vi "SPI IP.vi"() -> ()   [LabVIEW 2015]
uses:
  <userlib>/_NI SPI IP/FPGA/Controllers/Public/Transfer Settings.ctl
  <vilib>/Platform/TimedLoop/XDataNode/timing_clust.ctl
  <vilib>/Platform/TimedLoop/XDataNode/nitl_modes.ctl
  <vilib>/Platform/TimedLoop/XDataNode/wakeup.ctl
  <userlib>/_NI SPI IP/FPGA/Controllers/Public/Spi Master Inputs.ctl
  <vilib>/rvi/eio/common/nirviEmuTemplateMethod_errors.vi
  <vilib>/rvi/Emulation/niFpgaSctlEmulationGetInTimedLoop.vi
  <vilib>/rvi/Emulation/niFpgaEmulationReportErrorSimple.vi
  <vilib>/rvi/Emulation/niFpgaGetClockAttributes.vi
  <vilib>/rvi/Emulation/niFpgaCriticalErrorInLSC.vi
  SubVIs/Digital Logic/FPGA Simple PWM U32.vi
  <vilib>/eio/EIONode/EIONode.xnode
  <vilib>/Platform/TimedLoop/XDataNode/XDataNode.xnode
  <userlib>/_NI SPI IP/FPGA/Controllers/NI SPI IP FPGA.lvlib
  <vilib>/Platform/TimedLoop/XDataNode/XDNodeRunTimeDep.lvlib
panel:
  out "MOSI":bool
  out "Clock":bool
  out "Chip Select":bool
  in  "spi transfer settings":T1={"Divide Value"=20, "Transfer Length (bits)"=32, "CS Asserted Polarity"=FALSE, "Clock Polarity (CPOL)"=FALSE, "Clock Phase (CPHA)"=FALSE, "Lengthen MISO Setup"=FALSE, "Direction Change Bit"=0, "MOSI Starts as Output"=FALSE, "Tristatable MOSI"=FALSE} {"Direction Change Bit" max=64 step=1; "Transfer Length (bits)" min=1 max=64 step=1}
  in  "manual assert chip select":bool
  out "ready for input":bool
  out "read data":u64 format="%.0x"
  in  "data to write":u64 format="%.0x"
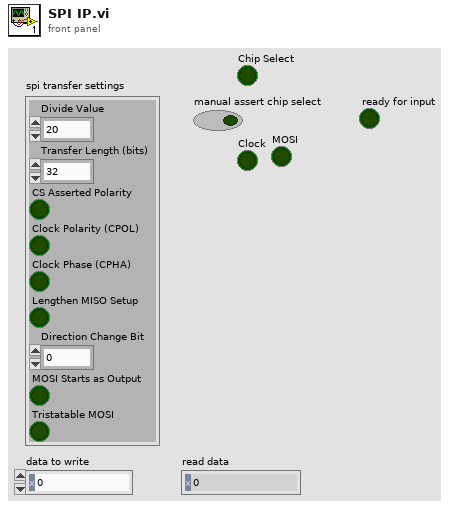
[diagram p1: front panel]
types:
  T1 = typedef "NI SPI IP FPGA.lvlib/Transfer Settings.ctl" = cluster{"Divide Value":u8, "Transfer Length (bits)":u8, "CS Asserted Polarity":bool, "Clock Polarity (CPOL)":bool, "Clock Phase (CPHA)":bool, "Lengthen MISO Setup":bool, "Direction Change Bit":u8, "MOSI Starts as Output":bool, "Tristatable MOSI":bool}
  T2 = typedef "NI SPI IP FPGA.lvlib/Spi Master Inputs.ctl" = cluster{"MISO":bool}
  T3 = typedef "XDNodeRunTimeDep.lvlib/timing_clust.ctl" = cluster{"Expected End [f-1]":u64, "Actual End [f-1]":u64, "Finished Late? [f-1]":bool, "Expected End [i-1]":u64, "Actual End [i-1]":u64, "Finished Late? [i-1]":bool, "Expected Start [i]":u64, "Actual Start [i]":u64, "Expected Start [f]":u64, "Actual Start [f]":u64, "Source Name":string, "Structure Name":string, "Period":i64, "Deadline":i64, "Offset":i64, "Start":i64, "Priority":i32, "Timeout":i32, "Mode":T4, "Wakeup Reason":T5, "Error":errorcluster, "Source Type":string, "Secondary Source Type":string, "Global End Time":u64, "Global Start Time":u64, "Frame Duration":u64, "Iteration Duration":u64, "Assigned CPU":i32, "I/O Scan Engine Mode":u32}
  T4 = typedef "XDNodeRunTimeDep.lvlib/nitl_modes.ctl" = enum32{"No Change", "Process missed periods, maintain original phase", "Discard missed periods, maintain original phase", "Process missed periods, ignore original phase", "Discard missed periods, ignore original phase"}
  T5 = typedef "XDNodeRunTimeDep.lvlib/wakeup.ctl" = enum32{"Normal", "Aborted", "Asynchronous wakeup", "Timing source error", "Timed loop error", "Timeout"}
  T6 = typedef "NI SPI IP FPGA.lvlib/Spi Master Outputs.ctl" = cluster{"Chip Select":bool, "Clock":bool, "MOSI":bool, "MOSI OE":bool}
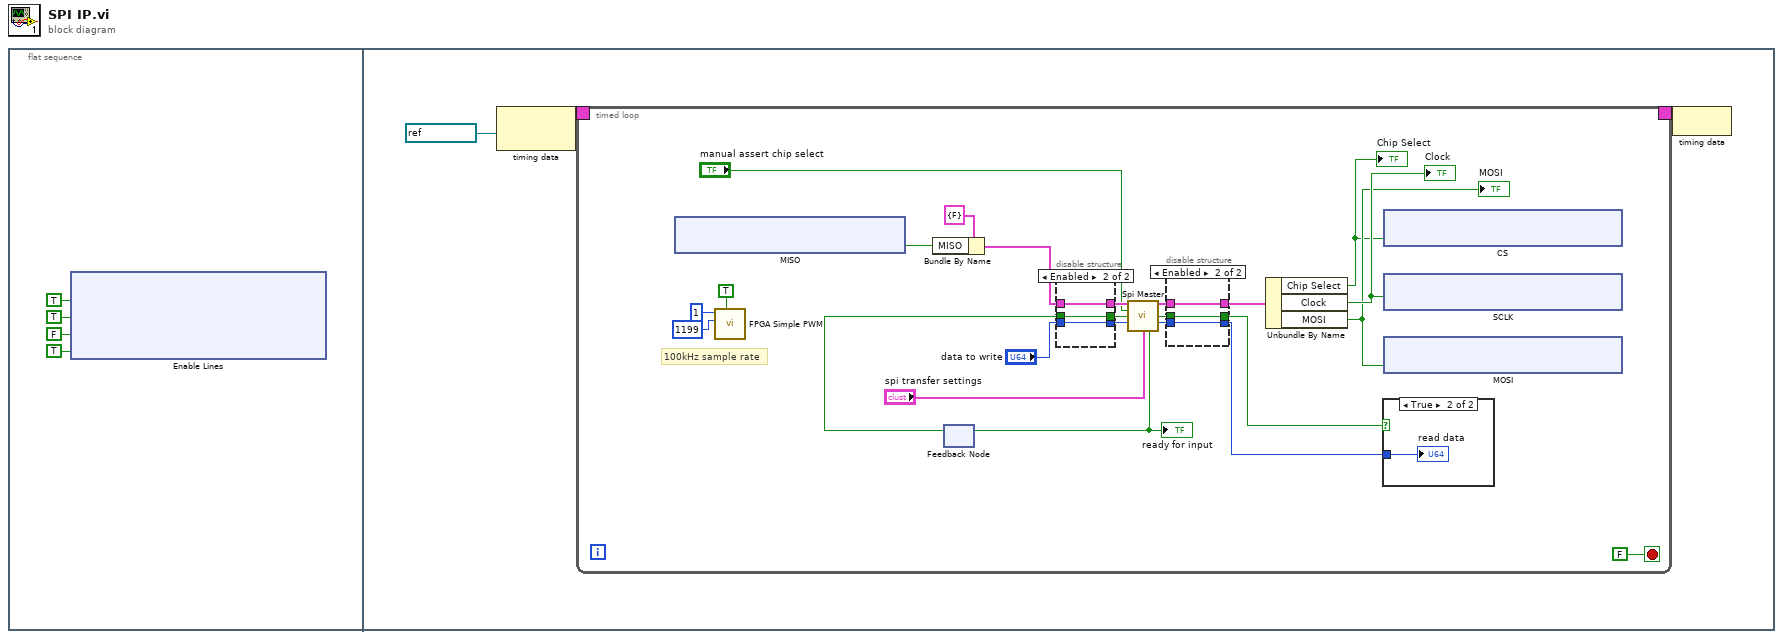
[diagram p0: block diagram]
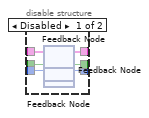
[diagram p2: hidden frame]
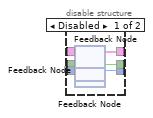
[diagram p3: hidden frame]
diagram:
  n1 = flat-sequence {
    frame #0 {
      n2 = xnode "Enable Lines"("sbRIO-9651 Socket\\PMOD1_Pin1_enable"=TRUE ("sbRIO-9651 Socket\\PMOD1_Pin1_enable"), "sbRIO-9651 Socket\\PMOD1_Pin2_enable"=TRUE ("sbRIO-9651 Socket\\PMOD1_Pin2_enable"), "sbRIO-9651 Socket\\PMOD1_Pin3_enable"=FALSE ("sbRIO-9651 Socket\\PMOD1_Pin3_enable"), "sbRIO-9651 Socket\\PMOD1_Pin4_enable"=TRUE ("sbRIO-9651 Socket\\PMOD1_Pin4_enable")) -> ()  [unwired: 4 in, 4 out]
    }
    frame #1 {
      n3 = node-c288(refnum<k21> "120MHz" ("Source Name")) -> (w7:T3)
      n4 = timed-loop {
        timing: w7 -> [_]
        timing-out: [_] -> w6
        stop <- FALSE stop-if-true
        # "100kHz sample rate"
        n5 = xnode "MISO"() -> ("sbRIO-9651 Socket\\PMOD1_Pin3_in"=w23:bool)  [unwired: 1 in, 1 out]
        n6 = call-poly "FPGA Simple PWM.vi"("PWM Enabled?"=TRUE, "Low Count"=u32 1199, "High Count"=u32 1) -> ()  [unwired: 8 in, 1 out]
        n7 = Bundle By Name(cluster=T2 {"MISO"=FALSE} ("spi input"), "MISO"=w23) -> (w28:T2)
        n8 = feedback #1() -> (w8:bool)  [unwired: 1 in]
        n9 = disable-structure shown="Enabled" {
          disable-tunnel: w28 -> [w46 w49]
          disable-tunnel: w8 -> [w45 w48]
          disable-tunnel: [w44 w47] -> w14
          disable-tunnel: [w43 w49] -> w13
          disable-tunnel: [w42 w48] -> w12
          disable-tunnel: "data to write" -> [w41 w47]
          frame Disabled {
            n10 = feedback #2() -> (w43:T2)  [unwired: 1 in]
            n11 = feedback-in #2(w46) -> ()
            n12 = feedback #3() -> (w42:bool)  [unwired: 1 in]
            n13 = feedback-in #3(w45) -> ()
            n14 = feedback #4() -> (w44:u64)  [unwired: 1 in]
            n15 = feedback-in #4(w41) -> ()
          }
          frame Enabled {
          }
        }
        n16 = call <userlib>:"Spi Master.vi"("spi input"=w13, "manual assert chip select"="manual assert chip select", "start strobe"=w12, "data to write"=w14, "spi transfer settings"="spi transfer settings") -> ("spi output"=w29:T6, "read data valid"=w27:bool, "read data"=w26:u64, "ready for input"=w20:bool)  [unwired: 7 in]
        "ready for input" <- w20
        n17 = feedback-in #1(w20) -> ()
        n18 = disable-structure shown="Enabled" {
          disable-tunnel: w29 -> [w37 w40]
          disable-tunnel: w27 -> [w36 w39]
          disable-tunnel: w26 -> [w35 w38]
          disable-tunnel: [w34 w38] -> w16
          disable-tunnel: [w33 w40] -> w15
          disable-tunnel: [w32 w39] -> w10
          frame Disabled {
            n19 = feedback #5() -> (w33:T6)  [unwired: 1 in]
            n20 = feedback-in #5(w37) -> ()
            n21 = feedback #6() -> (w32:bool)  [unwired: 1 in]
            n22 = feedback-in #6(w36) -> ()
            n23 = feedback #7() -> (w34:u64)  [unwired: 1 in]
            n24 = feedback-in #7(w35) -> ()
          }
          frame Enabled {
          }
        }
        n25 = Unbundle By Name(w15) -> ("Chip Select"=w24:bool, "Clock"=w30:bool, "MOSI"=w25:bool)
        "Chip Select" <- w24
        "Clock" <- w30
        "MOSI" <- w25
        n26 = case shown="True" w10 {
          tunnel: w16 -> [_ w50]
          frame False {
          }
          frame True {
            "read data" <- w50
          }
        }
        n27 = xnode "CS"("sbRIO-9651 Socket\\PMOD1_Pin1_out"=w24) -> ()  [unwired: 1 in, 1 out]
        n28 = xnode "SCLK"("sbRIO-9651 Socket\\PMOD1_Pin4_out"=w30) -> ()  [unwired: 1 in, 1 out]
        n29 = xnode "MOSI"("sbRIO-9651 Socket\\PMOD1_Pin2_out"=w25) -> ()  [unwired: 1 in, 1 out]
      }
      n30 = node-c288(w6) -> ()
    }
  }
